vi "Configure Modulation Control.vi"(0 "VISA resource name":refnum<visa-resource-name>, 5 "Modulation":u32(ring) items=["Not Available", "Available"], 7 "Control Input":u32(ring) items=["Disabled", "Control Voltage", "Control Current"], 9 "Modulation Type":u32(ring) items=["Multiplication", "Addition"], 11 "error in (no error)":errorcluster) -> (4 "VISA resource name out":refnum<visa-resource-name>, 15 "error out":errorcluster)   [LabVIEW 2022 SP3, in "MagnaDC.lvlib"]
uses:
  MagnaDC.lvlib
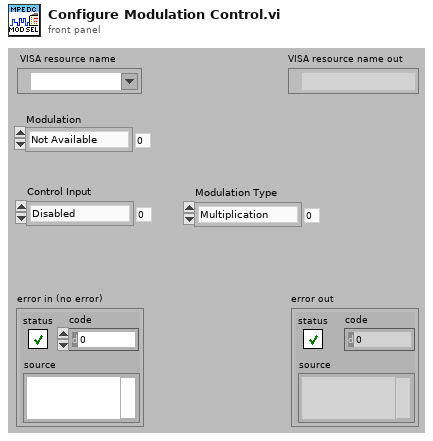
[diagram p1: front panel]
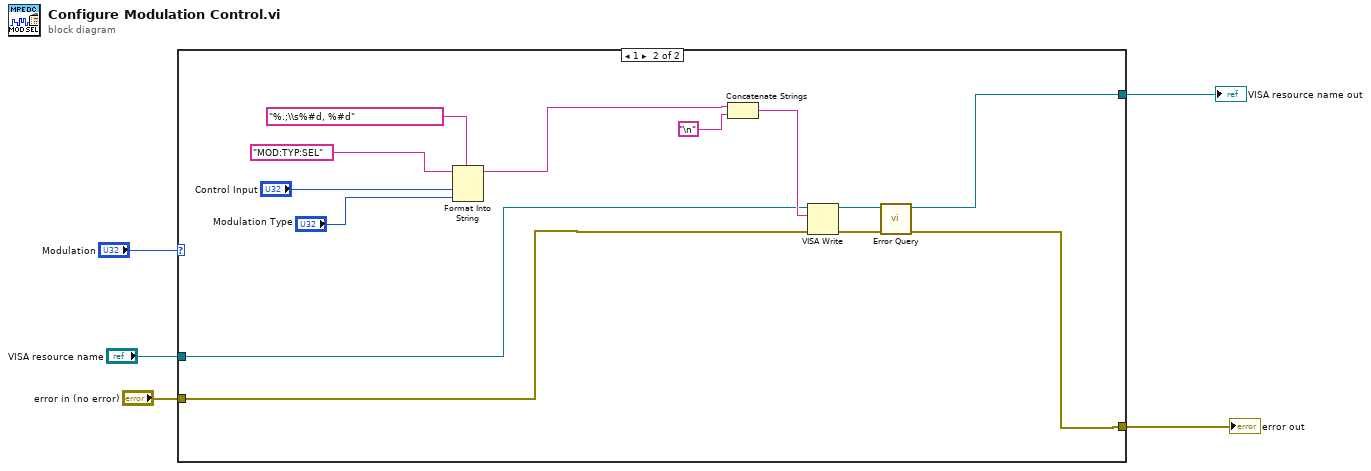
[diagram p0: block diagram]
diagram:
  n1 = case shown="1" "Modulation" {
    tunnel: "VISA resource name" -> [w6 w11]
    tunnel: "error in (no error)" -> [w7 w10]
    tunnel: [w6 w13] -> w2
    tunnel: [w7 w12] -> w1
    frame 0, Default {
    }
    frame 1 {
      n2 = Format Into String(format string="%.;\\s%#d, %#d", initial string="MOD:TYP:SEL", "Control Input", "Modulation Type") -> (resulting string=w14:string)  [unwired: 1 in, 1 out]
      n3 = Concatenate Strings(w14, "\n") -> (w15:string)
      n4 = VISA Write(VISA resource name=w11, write buffer=w15, error in (no error)=w10) -> (VISA resource name out=w18:refnum<visa-resource-name>, error out=w17:errorcluster)  [unwired: 1 out]
      n5 = call "Error Query.vi"("error in (no error)"=w17, "VISA resource name"=w18) -> ("error out"=w12:errorcluster, "VISA resource name out"=w13:refnum<visa-resource-name>)  [unwired: 6 in, 2 out]
    }
  }
  "error out" <- w1
  "VISA resource name out" <- w2
